vi "Set Schedule.vi"(8 "error in (no error)":errorcluster, 9 "Cron":refnum<class "Cron.lvclass">=refnum, 11 "module in":refnum<class "CRON.lvclass">) -> (0 "error out":errorcluster, 3 "module out":refnum<class "CRON.lvclass">, 4 "timed out?":bool)   [LabVIEW 2024, in "CRON.lvclass"]
uses:
  CRON.lvclass
  CRON.lvclass/CRON.ctl
  C:/Git/JA/JQMH/RQMHCore/ModuleCore/Module.lvclass
  C:/Git/JA/JQMH/ModuleTemplates/CRON/CRON.lvclass
  RQMHCore/ModuleCore/Module.lvclass
  RQMHCore/ModuleCore/Reply.ctl
  <vilib>/LabVIEW Open Source Project/Cron Scheduler/Cron/Cron.lvclass
  Set Schedule Args.ctl
  Set Schedule ReplyArgs.ctl
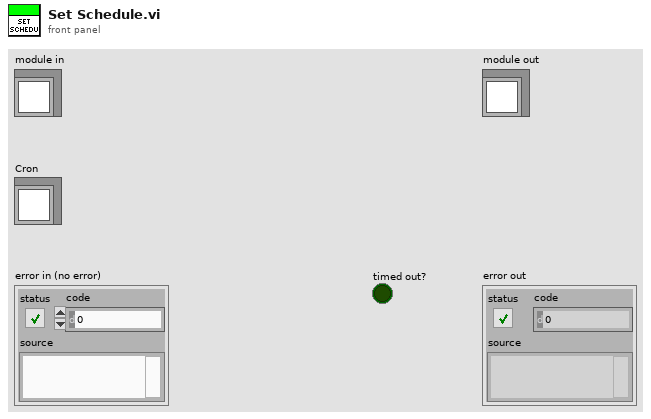
[diagram p1: front panel]
types:
  T1 = typedef "CRON.lvclass/Set Schedule Args.ctl" = cluster{"Cron":refnum<class "Cron.lvclass">}
  T2 = typedef "Module.lvclass/Reply.ctl" = cluster{"Expects Reply":bool, "Reply":refnum<notifier>}
  T3 = typedef "CRON.lvclass/Set Schedule ReplyArgs.ctl" = cluster{"null":bool}
  T4 = cluster{"RQMH_REPLYARGS":T3, "error in (no error)":errorcluster}
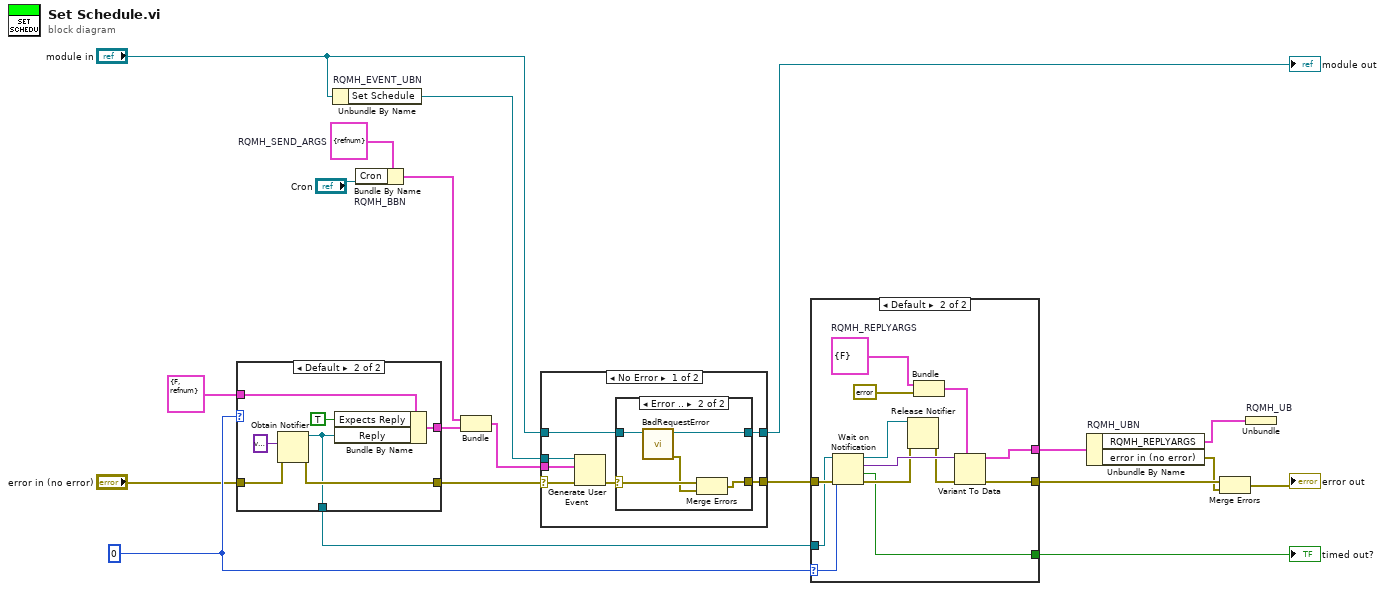
[diagram p0: block diagram]
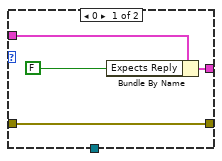
[diagram p4: hidden frame]
diagram:
  w13 = 0 ("timeout in ms (-1)")
  w10 = T1 {"Cron"=refnum}  # RQMH_SEND_ARGS
  n1 = case shown="Default" w13 {
    tunnel: [w23 w30] -> w20
    tunnel: "error in (no error)" -> [w21 w29]
    tunnel: [w21 w28] -> w18
    tunnel: [_ w27] -> w16
    tunnel: T2 {"Expects Reply"=FALSE, "Reply"=refnum} ("Reply") -> [w24 w26]
    frame 0 {
      n2 = Bundle By Name(cluster=w24, "Expects Reply"=FALSE) -> (w23:T2)
    }
    frame Default {
      n3 = Obtain Notifier(notification data type=variant, error in (no error)=w29) -> (notifier out=w27:refnum<notifier>, error out=w28:errorcluster)  [unwired: 2 in, 1 out]
      n4 = Bundle By Name(cluster=w26, "Expects Reply"=TRUE, "Reply"=w27) -> (w30:T2)
    }
  }
  n5 = Unbundle By Name "RQMH_EVENT_UBN"("module in") -> ("Set Schedule"=w8:refnum<user-event>)
  n6 = Bundle By Name "RQMH_BBN"(cluster=w10, "Cron"="Cron") -> (w7:T1)
  n7 = Bundle("RQMH_SEND_ARGS"=w7, "Reply"=w20) -> (w19:cluster{"RQMH_SEND_ARGS":T1, "Reply":T2})  [unwired: 1 in]
  n8 = case shown="No Error" w18 {
    selector: w18 -> [w35 w46]
    tunnel: w19 -> [w38 _]
    tunnel: w8 -> [w37 _]
    tunnel: [w34 w46] -> w17
    tunnel: "module in" -> [w33 w47]
    tunnel: [w32 w47] -> w11
    frame No Error {
      n9 = Generate User Event(user event=w37, event data cluster=w38, error in=w35) -> (error out=w36:errorcluster)  [unwired: 1 in, 1 out]
      n10 = case shown="Error .." w36 {
        selector: w36 -> [w39 w45]
        tunnel: [w39 w44] -> w34
        tunnel: w33 -> [w40 w43]
        tunnel: [w40 w42] -> w32
        frame No Error {
        }
        frame Error {
          n11 = call "BadRequestError.vi"("JQMHModule in"=w43) -> ("error out"=w41:errorcluster, "JQMHModule out"=w42:refnum<class "CRON.lvclass">)  [unwired: 9 in]
          n12 = Merge Errors(w45, w41) -> (w44:errorcluster)
        }
      }
    }
    frame Error {
    }
  }
  "module out" <- w11
  n13 = case shown="Default" w13 {
    selector: w13 -> [_ w52]
    tunnel: w17 -> [w48 w61]
    tunnel: w16 -> [_ w60]
    tunnel: [_ w53] -> w15
    tunnel: [w48 w50] -> w6
    tunnel: [_ w49] -> w5
    frame 0 {
    }
    frame Default {
      w51 = T3 {"null"=FALSE}  # RQMH_REPLYARGS
      n14 = Wait on Notification(notifier=w60, timeout in ms (-1)=w52, error in (no error)=w61) -> (notifier out=w56:refnum<notifier>, notification=w57:variant, timed out?=w53:bool, error out=w55:errorcluster)  [unwired: 1 in]
      n15 = Release Notifier(notifier=w56, error in (no error)=w55) -> (error out=w54:errorcluster)  [unwired: 1 in, 2 out]
      n16 = Bundle("RQMH_REPLYARGS"=w51, "error in (no error)"=errorcluster {"status"=FALSE, "code"=0, "source"=""}) -> (w59:T4)  [unwired: 1 in]
      n17 = Variant To Data(error in=w54, type=w59, Variant=w57) -> (data=w49:T4, error out=w50:errorcluster)
    }
  }
  "timed out?" <- w15
  n18 = Unbundle By Name "RQMH_UBN"(w5) -> ("RQMH_REPLYARGS"=w2:T3, "error in (no error)"=w3:errorcluster)
  n19 = Merge Errors(w6, w3) -> (→"error out":errorcluster)
  n20 = Unbundle "RQMH_UB"(w2) -> ()  [unwired: 1 out]
